vi "camera_lightswitchCF3.vi"() -> ()   [LabVIEW 2017]
uses:
  <vilib>/vision/driver/NI_Vision_Acquisition_Software.lvlib
panel:
  out "Lights ON?":bool
  out "Lights OFF?":bool
  in  "Lights ON":timestamp=timestamp(57600 s since 1904-01-01) format="%<%X>T"
  in  "Lights OFF":timestamp=timestamp(14400 s since 1904-01-01) format="%<%X>T"
  in  "Shutter speed dark":dbl(slide)=0.125 min=0.0 max=0.25 scale=0.0..0.25
  in  "Gain dark":dbl(slide) scale=0.0..20.5
  in  "Brightness dark":dbl(slide) min=-20.0 max=20.0 step=0.5 scale=-20.0..20.0
  in  "Save Images":bool
  in  "Shutter speed light":dbl(slide)=0.125 min=0.0 max=0.25 scale=0.0..0.25
  in  "Path":path=path "C:/Users/MaloofLab/Desktop/photos/test"
  in  "Gain light":dbl(slide) scale=0.0..20.5
  in  "Image Count":i16
  in  "Brightness light":dbl(slide) min=-20.0 max=20.0 step=0.5 scale=-20.0..20.0
  out "IR LED Status":bool
  out "Last Time-lapse image":T1(plugin-control)
  out "Current Time":string
  out "Next snapshot at:":string
  in  "Time-lapse interval":dbl=900.0 format="%<%H:%M:%S>t"
  out "Live":T1(plugin-control)
  in  "?":bool
  in  "Camera Name":string="cam1"
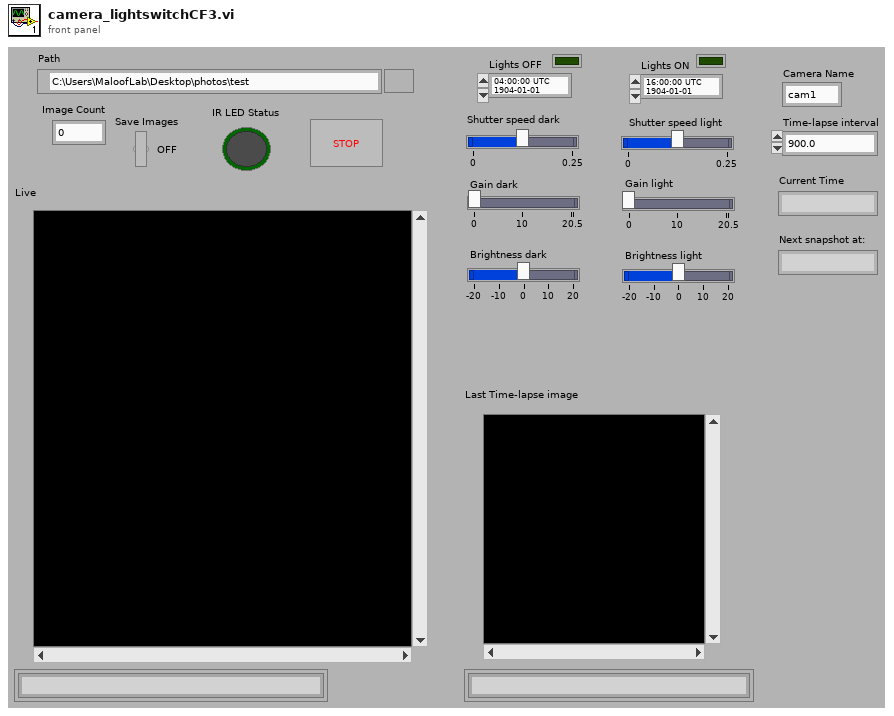
[diagram p1: front panel]
types:
  T1 = typedef "IMAQ Image.ctl" = refnum<image>
  T2 = typedef "IMAQdx.ctl" = refnum<k21>
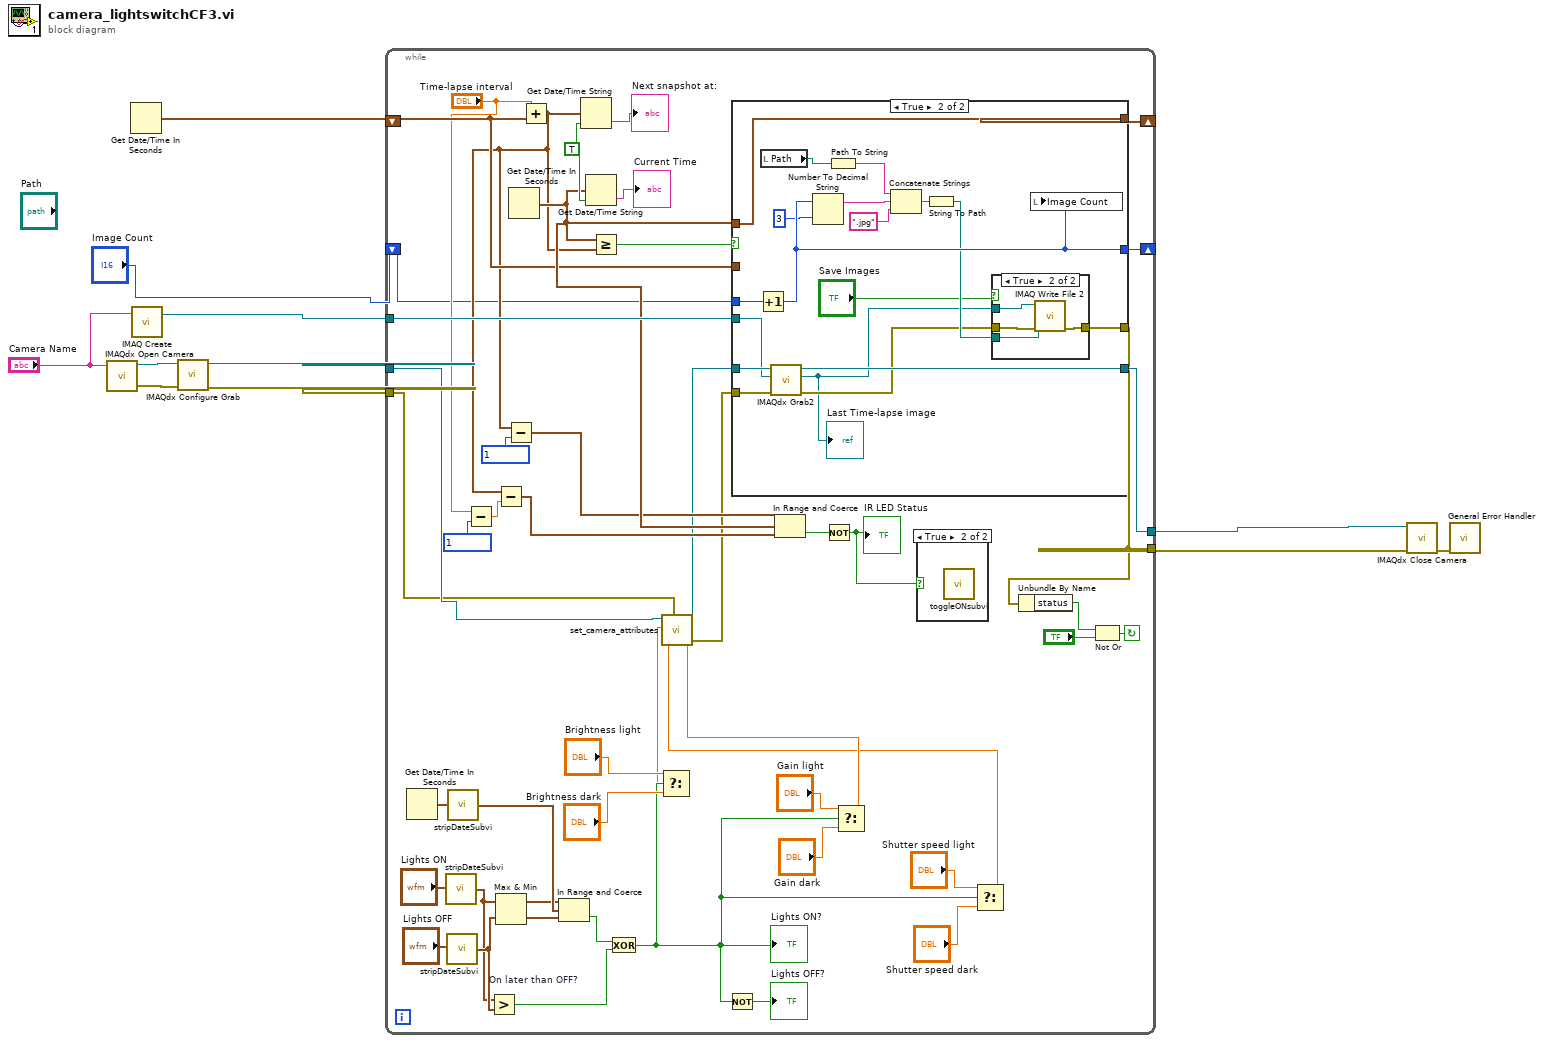
[diagram p0: block diagram]
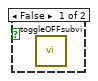
[diagram p2: hidden frame]
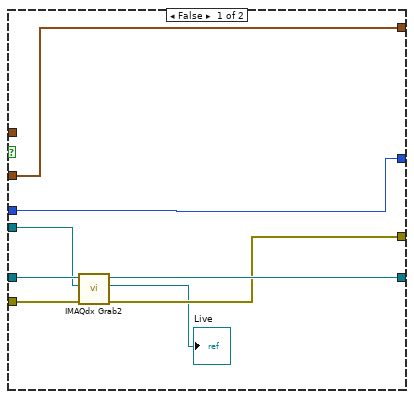
[diagram p3: hidden frame]
diagram:
  n1 = call <vilib>:"IMAQdx Open Camera.vi"("Session In"="Camera Name") -> ("error out"=w11:errorcluster, "Session Out"=w10:T2)  [unwired: 9 in]
  n2 = Get Date/Time In Seconds() -> (seconds since 1Jan1904=w3:timestamp)
  n3 = call "IMAQ Create"("Image Name"="Camera Name") -> ("New Image"=w7:T1)  [unwired: 4 in, 1 out]
  n4 = call <vilib>:"IMAQdx Configure Grab.vi"("error in"=w11, "Session In"=w10) -> ("error out"=w9:errorcluster, "Session Out"=w8:T2)  [unwired: 8 in]
  n5 = while {
    tunnel: w9 -> [w17]
    tunnel: w8 -> [w18]
    tunnel: w7 -> [w53]
    tunnel: [w52] -> w6
    tunnel: [w51] -> w5
    shift-right: [w54] -> _
    shift-left: w3 -> [w48]
    shift-right: [w38] -> _
    shift-left: "Image Count" -> [w39]
    stop <- w60 continue-if-true
    w55 = TRUE
    n6 = Get Date/Time In Seconds() -> (seconds since 1Jan1904=w26:timestamp)
    n7 = call "stripDateSubvi.vi"("Time Stamp"="Lights ON") -> ("Time Stamp 2"=w21:timestamp)
    n8 = call "stripDateSubvi.vi"("Time Stamp"="Lights OFF") -> ("Time Stamp 2"=w22:timestamp)
    n9 = call "stripDateSubvi.vi"("Time Stamp"=w26) -> ("Time Stamp 2"=w25:timestamp)
    n10 = Subtract(x="Time-lapse interval", y=1) -> (x-y=w42:dbl)
    n11 = Greater? "On later than OFF?"(x=w21, y=w22) -> (0:w35:bool)
    n12 = Max & Min(x=w21, y=w22) -> (max(x,y)=w20:timestamp, min(x,y)=w19:timestamp)
    n13 = Get Date/Time In Seconds() -> (seconds since 1Jan1904=w49:timestamp)
    n14 = Add(x="Time-lapse interval", y=w48) -> (x+y=w47:timestamp)
    n15 = Subtract(x=w47, y=w42) -> (x-y=w46:timestamp)
    n16 = Subtract(x=w47, y=1) -> (x-y=w45:timestamp)
    n17 = In Range and Coerce(upper limit=w20, x=w25, lower limit=w19) -> (In Range?=w36:bool)  [unwired: 1 out]
    n18 = Get Date/Time String(seconds (now)=w47, want seconds? (F)=w55) -> (time string=→"Next snapshot at:":string)  [unwired: 1 in, 1 out]
    n19 = Get Date/Time String(seconds (now)=w49, want seconds? (F)=w55) -> (time string=→"Current Time":string)  [unwired: 1 in, 1 out]
    n20 = Greater Or Equal?(x=w49, y=w47) -> (x >= y?=w37:bool)
    n21 = Exclusive Or(1:w35, 2:w36) -> (0:w27:bool)
    "Lights ON?" <- w27
    n22 = Select(t="Brightness light", s=w27, f="Brightness dark") -> (s? t:f=w14:dbl)
    n23 = Not(x=w27) -> (.not. x?=→"Lights OFF?":bool)
    n24 = In Range and Coerce(upper limit=w45, x=w49, lower limit=w46) -> (In Range?=w44:bool)  [unwired: 1 out]
    n25 = Not(x=w44) -> (.not. x?=w40:bool)
    "IR LED Status" <- w40
    n26 = Select(t="Gain light", s=w27, f="Gain dark") -> (s? t:f=w13:dbl)
    n27 = case shown="True" w40 {
      frame False {
        n28 = call "toggleOFFsubvi.vi"() -> ()  [unwired: 2 in]
      }
      frame True {
        n29 = call "toggleONsubvi.vi"() -> ()  [unwired: 2 in]
      }
    }
    n30 = Select(t="Shutter speed light", s=w27, f="Shutter speed dark") -> (s? t:f=w12:dbl)
    n31 = call "set_camera_attributes.vi"("Session In"=w18, "Brightness"=w14, "Gain"=w13, "Shutter"=w12, "error in (no error)"=w17) -> ("Session Out"=w16:T2, "error out"=w15:errorcluster)  [unwired: 1 in]
    n32 = case shown="True" w37 {
      tunnel: w49 -> [_ w77]
      tunnel: w48 -> [w68 _]
      tunnel: [w68 w77] -> w54
      tunnel: w53 -> [w65 w85]
      tunnel: w16 -> [w66 w86]
      tunnel: w15 -> [w67 w84]
      tunnel: [w64 w83] -> w52
      tunnel: [w63 w73] -> w51
      tunnel: w39 -> [w61 w78]
      tunnel: [w61 w75] -> w38
      frame False {
        n33 = call <vilib>:"IMAQdx Grab2.vi"("error in"=w67, "Image In"=w65, "Session In"=w66) -> ("error out"=w63:errorcluster, "Image Out"=→"Live":T1, "Session Out"=w64:T2)  [unwired: 5 in, 1 out]
      }
      frame True {
        n34 = Increment(x=w78) -> (x+1=w75:i16)
        n35 = local read "Path"() -> (w76:path)
        n36 = call <vilib>:"IMAQdx Grab2.vi"("error in"=w84, "Image In"=w85, "Session In"=w86) -> ("error out"=w71:errorcluster, "Image Out"=w70:T1, "Session Out"=w83:T2)  [unwired: 5 in, 1 out]
        "Last Time-lapse image" <- w70
        n37 = Number To Decimal String(number=w75, width (-)=i16 3) -> (decimal integer string=w80:string)
        n38 = Path To String(path=w76) -> (string=w81:string)
        n39 = Concatenate Strings(w81, w80, ".jpg" ("string")) -> (w82:string)
        n40 = String To Path(string=w82) -> (path=w72:path)
        n41 = case shown="True" "Save Images" {
          tunnel: [w87 w91] -> w73
          tunnel: w72 -> [_ w90]
          tunnel: w71 -> [w87 w89]
          tunnel: w70 -> [_ w88]
          frame False {
          }
          frame True {
            n42 = call-poly "IMAQ Write File 2"("error in (no error)"=w89, "File Path"=w90, "Image"=w88) -> ("error out"=w91:errorcluster)  [unwired: 7 in, 1 out]
          }
        }
        n43 = local write "Image Count"(w75) -> ()
      }
    }
    n44 = Unbundle By Name(w51) -> ("status"=w58:bool)
    n45 = Not Or(1:"?", 2:w58) -> (0:w60:bool)
  }
  n46 = call <vilib>:"IMAQdx Close Camera.vi"("error in"=w5, "Session In"=w6) -> ("error out"=w4:errorcluster)  [unwired: 9 in]
  n47 = call <vilib>:"General Error Handler.vi"("error in (no error)"=w4) -> ()  [unwired: 10 in, 5 out]
